vi "FTW-ERR-UnknownJob.vi"(8 "error in":errorcluster, 10 "Unknown Job":string) -> (0 "error out":errorcluster)   [LabVIEW 2013]
doc: "Toto, I've a feeling we're not in Kansas any more.... We must be over the rainbow!"
panel:
  # "Inputs"
  # "Outputs"
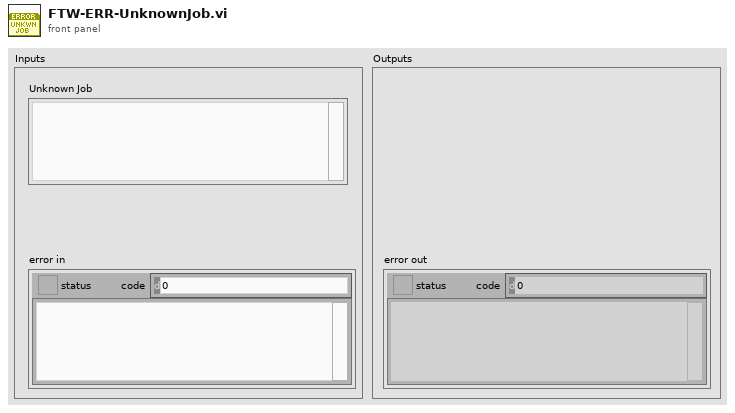
[diagram p1: front panel]
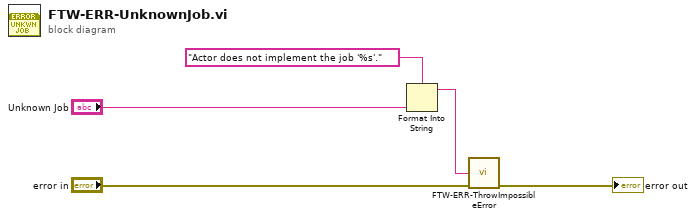
[diagram p0: block diagram]
diagram:
  n1 = Format Into String(format string="Actor does not implement the job '%s'.", "Unknown Job") -> (resulting string=w1:string)  [unwired: 2 in, 1 out]
  n2 = call "FTW-ERR-ThrowImpossibleError.vi"("Reason this error should never happen"=w1, "error in"="error in") -> ("error out"=→"error out":errorcluster)  [unwired: 13 in]
